vi "Digital IO to Plot.vi"(10 "Boolean Value":bool, 11 "Multiplier":u16) -> (3 "Output":u16)   [LabVIEW 2023]
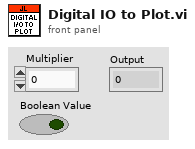
[diagram p1: front panel]
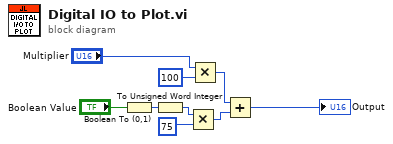
[diagram p0: block diagram]
diagram:
  n1 = Boolean To (0,1)(Boolean="Boolean Value") -> (0, 1=w2:i16)
  n2 = To Unsigned Word Integer(number=w2) -> (unsigned 16bit integer=w1:u16)
  n3 = Multiply(x=w1, y=u16 75) -> (x*y=w5:u16)
  n4 = Multiply(x="Multiplier", y=u16 100) -> (x*y=w8:u16)
  n5 = Add(x=w8, y=w5) -> (x+y=→"Output":u16)
